vi "Load Limits From Sequence File.vi"(0 "Test Number and Bin Generator":refnum<class "Test Number and Bin Generator.lvclass">=refnum, 11 "error in (no error)":errorcluster) -> (4 "Test Number and Bin Generator 2":refnum<class "Test Number and Bin Generator.lvclass">, 8 "Evaluations From Sequence File":T1[](array[typedef]) {"Low Limit" format="%#_13g"; "SI Scaling" items=["femto"=-15, "pico"=-12, "nano"=-9, "micro"=-6, "milli"=-3, "percent"=-2, ""=0, "kilo"=3, "mega"=6, "giga"=9, "tera"=12]}, 15 "error out":errorcluster)   [LabVIEW 2018, in "Test Number and Bin Generator.lvlib" / "Test Number and Bin Generator.lvclass"]
uses:
  Test Number and Bin Generator.lvclass
  Plugins/TestStand API Tools (TSAT).lvlibp/Evaluation Actions/Includes/Controls/TSAT Evaluation.ctl
  Plugins/TestStand API Tools (TSAT).lvlibp/Evaluation Actions/Includes/Controls/TSAT Eval SI Unit Scaling.ctl
  Plugins/TestStand API Tools (TSAT).lvlibp/Evaluation Actions/Includes/Controls/TSAT Evaluation Type.ctl
  Test Number and Bin Generator.lvclass/Test Number and Bin Generator.ctl
  Plugins/TestStand API Tools (TSAT).lvlibp/TSAT Examples/TSAT Examples.lvlib
  Plugins/TestStand API Tools (TSAT).lvlibp/Evaluation Actions/TSAT Evaluation Actions.lvlib
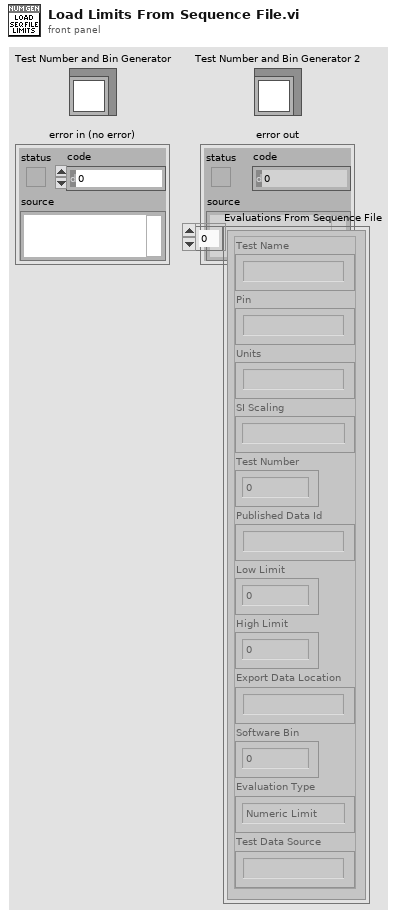
[diagram p1: front panel]
types:
  T1 = typedef "TestStand API Tools (TSAT).lvlibp/TSAT Evaluation Actions.lvlib/TSAT Evaluation.ctl" = cluster{"Test Name":string, "Pin":string, "Units":string, "SI Scaling":T2, "Test Number":i32, "Published Data Id":string, "Low Limit":dbl, "High Limit":dbl, "Export Data Location":string, "Software Bin":i64, "Evaluation Type":T3, "Test Data Source":string}
  T2 = typedef "TestStand API Tools (TSAT).lvlibp/TSAT Evaluation Actions.lvlib/TSAT Eval SI Unit Scaling.ctl" = i16
  T3 = typedef "TestStand API Tools (TSAT).lvlibp/TSAT Evaluation Actions.lvlib/TSAT Evaluation Type.ctl" = enum16{"Numeric Limit", "Pass/Fail", "None"}
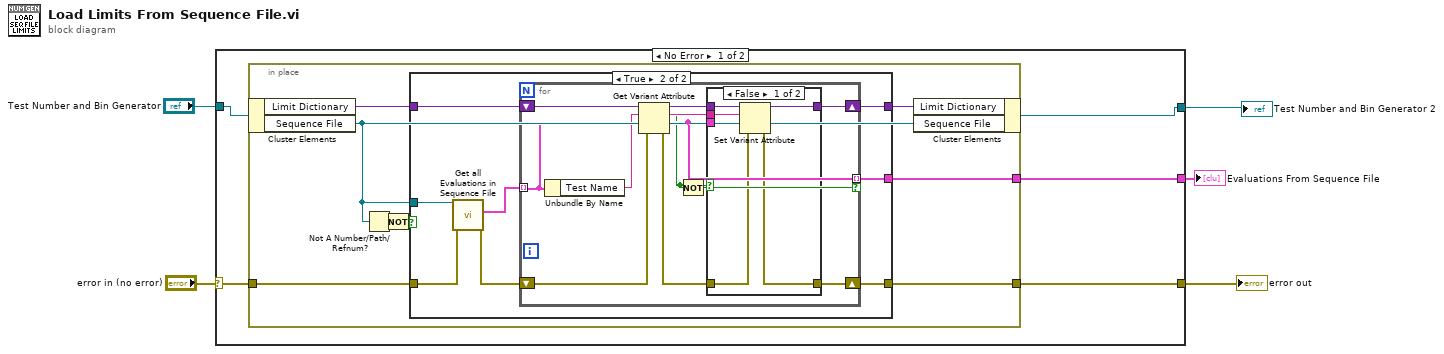
[diagram p0: block diagram]
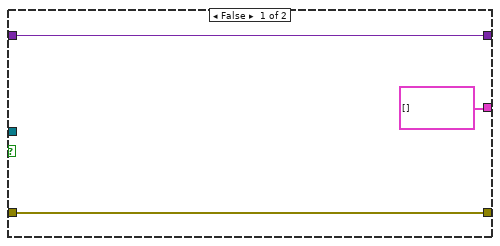
[diagram p2: hidden frame]
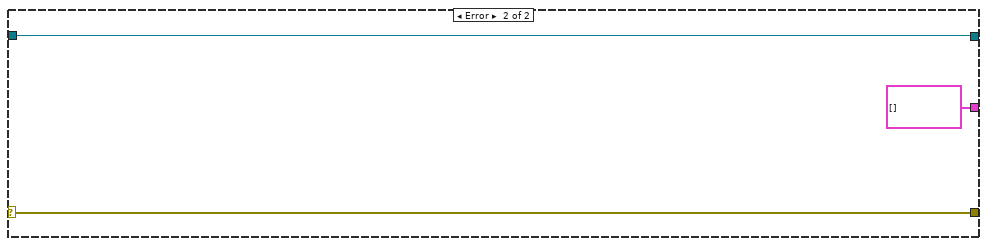
[diagram p4: hidden frame]
diagram:
  n1 = case shown="No Error" "error in (no error)" {
    selector: "error in (no error)" -> [w8 w49]
    tunnel: [w10 w49] -> w5
    tunnel: [w7 w50] -> w3
    tunnel: "Test Number and Bin Generator" -> [w9 w50]
    tunnel: [w6 T1[] []] -> w1
    frame No Error {
      n2 = in-place {
        in-place-border: [w15] -> w10
        in-place-border: w8 -> [w17]
        in-place-border: [w11] -> w6
        n3 = in-place-cluster #1(w9) -> ("Limit Dictionary"=w18:variant, "Sequence File"=w12:refnum<k7>)
        n4 = Not A Number/Path/Refnum?(number/path/refnum=w12) -> (NaN/Path/Refnum?=w14:bool)
        n5 = Not(x=w14) -> (.not. x?=w13:bool)
        n6 = case shown="True" w13 {
          tunnel: w18 -> [w21 w29]
          tunnel: w17 -> [w20 w24]
          tunnel: [w21 w28] -> w16
          tunnel: [w20 w27] -> w15
          tunnel: w12 -> [_ w26]
          tunnel: [T1[] [] w22] -> w11
          frame False {
          }
          frame True {
            n7 = call "Get all Evaluations in Sequence File.vi"("Error In"=w24, "Sequence File In"=w26) -> ("Error Out"=w23:errorcluster, "Evaluation Array"=w25:T1[])  [unwired: 7 in, 1 out]
            n8 = for {
              shift-right: [w36] -> w28
              shift-left: w29 -> [w39]
              tunnel: w25 -> [w32] mode=indexing
              shift-right: [w35] -> w27
              shift-left: w23 -> [w37]
              tunnel: [w32] -> w22 mode=indexing if=w30
              n9 = Unbundle By Name(w32) -> ("Test Name"=w33:string)
              n10 = Get Variant Attribute(Variant=w39, name=w33, error in=w37) -> (duplicate Variant=w38:variant, found=w31:bool, error out=w34:errorcluster)  [unwired: 1 in, 1 out]
              n11 = Not(x=w31) -> (.not. x?=w30:bool)
              n12 = case shown="False" w31 {
                tunnel: w38 -> [w45 w47]
                tunnel: [w44 w47] -> w36
                tunnel: [w41 w46] -> w35
                tunnel: w34 -> [w43 w46]
                tunnel: w33 -> [w42 _]
                tunnel: w32 -> [w40 _]
                frame False {
                  n13 = Set Variant Attribute(Variant=w45, name=w42, value=w40, error in=w43) -> (Variant out=w44:variant, error out=w41:errorcluster)  [unwired: 1 out]
                }
                frame True {
                }
              }
            }
          }
        }
        n14 = in-place-cluster #1("Limit Dictionary"=w16, "Sequence File"=w12) -> (w7:refnum<class "Test Number and Bin Generator.lvclass">)
      }
    }
    frame Error {
    }
  }
  "error out" <- w5
  "Test Number and Bin Generator 2" <- w3
  "Evaluations From Sequence File" <- w1
